vi "Get Number VS Speeds.vi"(11 "speeds":i32) -> (2 "function return":u32, 3 "speeds out":i32)   [LabVIEW 2018, in "AndorSDK.lvlib"]
doc: "EXPNETTYPE unsigned int WINAPI GetNumberVSSpeeds(int * speeds);"
uses:
  AndorSDK.lvlib
  ATMCD32D.dll
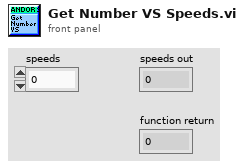
[diagram p1: front panel]
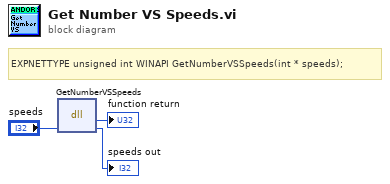
[diagram p0: block diagram]
diagram:
  # "EXPNETTYPE unsigned int WINAPI GetNumberVSSpeeds(int * speeds);"
  n1 = dll-call lib="PTH2babs E\nPersönliches02 - Arbeit03-HiwijobsLabviewCodelibANDOR\tAndor SDK\nATMCD32D.*" fn="GetNumberVSSpeeds"("speeds"="speeds") -> (→"function return":u32, "speeds"=→"speeds out":i32)  [unwired: 3 in, 2 out]
